vi "ReadFifo.vi"(8 "error in (no error)":errorcluster, 10 "N":i32, 11 "FPGA_Sim in":refnum<class "FPGA_Mock.lvclass">) -> (0 "error out":errorcluster, 2 "Data":dbl[](array[numeric]), 3 "FPGA_Sim out":refnum<class "FPGA_Mock.lvclass">)   [LabVIEW 2019, in "FPGA_Mock.lvclass"]
uses:
  FPGA_Mock.lvclass
  FPGA_Mock.lvclass/FPGA_Mock.ctl
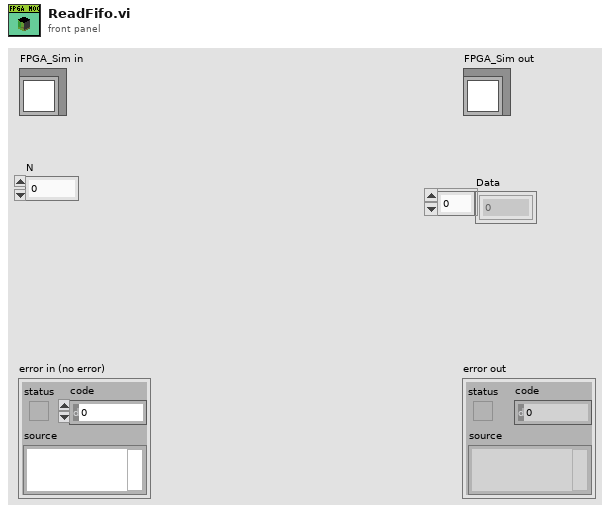
[diagram p1: front panel]
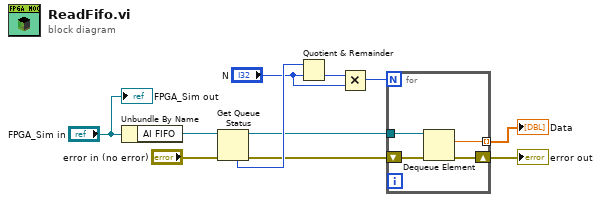
[diagram p0: block diagram]
diagram:
  n1 = Unbundle By Name("FPGA_Sim in") -> ("AI FIFO"=w10:refnum<queue>)
  n2 = Get Queue Status(queue=w10, error in (no error)="error in (no error)") -> (queue out=w5:refnum<queue>, error out=w2:errorcluster, # elements in queue=w9:i32)  [unwired: 1 in, 5 out]
  n3 = Quotient & Remainder(x=w9, y="N") -> (floor(x/y)=w8:i32)  [unwired: 1 out]
  n4 = Multiply(x=w8, y="N") -> (x*y=w6:i32)
  n5 = for {
    N: w6 -> [_]
    tunnel: w5 -> [w15]
    tunnel: [w14] -> w4 mode=indexing
    shift-right: [w12] -> w1
    shift-left: w2 -> [w13]
    n6 = Dequeue Element(queue=w15, error in (no error)=w13) -> (element=w14:dbl, error out=w12:errorcluster)  [unwired: 1 in, 2 out]
  }
  "error out" <- w1
  "Data" <- w4
  "FPGA_Sim out" <- "FPGA_Sim in"
